vi "Motor Velocity PID.vi"(5 "T_d":dbl=0.01, 6 "DC current max":dbl=0.437, 7 "T_i":dbl=inf, 9 "ccw velocity process variable":dbl[](array[numeric])=[0.0, 0.0, 0.0], 10 "ccw velocity setpoint":dbl[](array[numeric])=[0.0, 0.0, 0.0], 11 "K_p":dbl=0.008) -> (2 "DC current output":dbl[](array[numeric]))   [LabVIEW 2015]
uses:
  <vilib>/Simulation/Implementation/Shared/SIMSCR Execution Mode.ctl
  <vilib>/Simulation/Scripting/Companion Diagram/SimConfigNode/SimParams.ctl
  <vilib>/Simulation/Scripting/Companion Diagram/SimConfigNode/_simSolvers.ctl
  <vilib>/Simulation/Param Hierarchy/Typedefs/SIMPH Param Control Actions.ctl
  <vilib>/Simulation/Implementation/Shared/SIM limit type.ctl
  <vilib>/Simulation/Implementation/Shared/NILVSim_ParamChanged.vi
  <vilib>/Simulation/Implementation/Shared/NILVSIM_BeginStep.vi
  <vilib>/Simulation/ContinuousLinear/Implementation/NILVSim Derivative.llb/SIM derivative (vector).vi
  <vilib>/Simulation/ContinuousLinear/Implementation/NILVSim Integrator new.llb/SIM Integrator Distributor (vector).vi
  <vilib>/Simulation/ContinuousLinear/Implementation/NILVSim Integrator new.llb/SIM Integrator Collector (vector).vi
  <vilib>/Simulation/SignalArithmetic/Implementation/NILVSim Gain.llb/SIM Gain (vector,ScalarGain).vi
  <vilib>/Simulation/Nonlinear/Implementation/NILVSim Saturation.llb/SIM Saturation (vector).vi
  <vilib>/Simulation/Implementation/Shared/NILVSim_Manager.vi
  <vilib>/Utility/error.llb/Clear Errors.vi
  <vilib>/Simulation/Implementation/Shared/NILVSim_FinalizeModel.vi
  <vilib>/Simulation/Implementation/Shared/SIM Unbundle Sim Info.vi
  <vilib>/Simulation/Implementation/Shared/SIMSH Read Queue.vi
  <vilib>/Simulation/Implementation/Shared/NILVSim_Initialize.vi
  <vilib>/Simulation/Utility/Implementation/NILVSim Get Time and IsAcceptedStep.vi
  <vilib>/Simulation/Implementation/Shared/NILVSim_GetModelError.vi
  <vilib>/Simulation/Implementation/Shared/SIM SimErrorHandler.vi
  <vilib>/Simulation/Implementation/Shared/SIM Bundle Sim Info.vi
  <vilib>/Simulation/Scripting/Companion Diagram/SimConfigNode/SimDog.xnode
  <vilib>/Simulation/Implementation/XNodeFramework/SimXNode/SimX.xnode
  <vilib>/Simulation/ContinuousLinear/Implementation/NILVSim Integrator new.llb/SIM Integrator (vector).vi
  <vilib>/Simulation/Implementation/Shared/NI_SIM_Implementation.lvlib
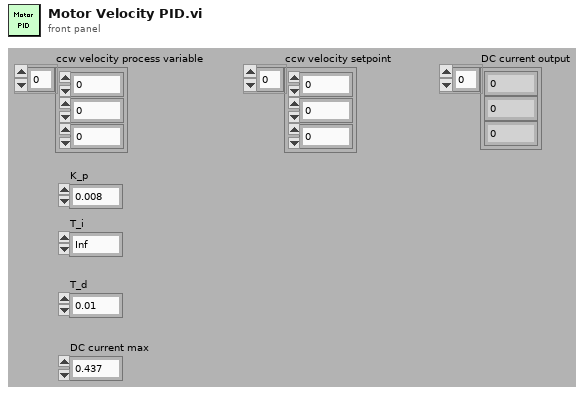
[diagram p1: front panel]
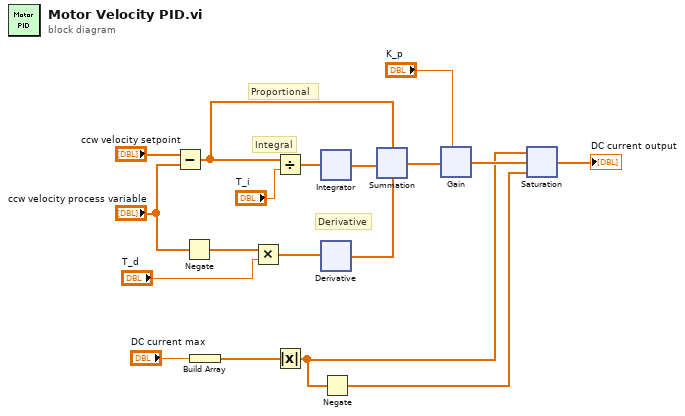
[diagram p0: block diagram]
diagram:
  # "Derivative"
  # "Integral"
  # "Proportional"
  n1 = Subtract(x="ccw velocity setpoint", y="ccw velocity process variable") -> (x-y=w12:dbl[])
  n2 = Negate(x="ccw velocity process variable") -> (-x=w10:dbl[])
  n3 = Build Array("DC current max") -> (w3:dbl[])
  n4 = Multiply(x=w10, y="T_d") -> (x*y=w8:dbl[])
  n5 = Divide(x=w12, y="T_i") -> (x/y=w18:dbl[])
  n6 = Absolute Value(x=w3) -> (abs(x)=w2:dbl[])
  n7 = xnode ("Integrator")("input"=w18) -> ("output"=w16:dbl[])  [unwired: 9 in, 2 out]
  n8 = xnode ("Derivative")("input"=w8) -> ("output"=w7:dbl[])  [unwired: 2 in]
  n9 = Negate ("Negate 2")(x=w2) -> (-x=w1:dbl[])
  n10 = xnode ("Summation")("Operand1"=w12, "Operand2"=w16, "Operand3"=w7) -> ("Result"=w15:dbl[])
  n11 = xnode ("Gain")("gain"="K_p", "input"=w15) -> ("output"=w6:dbl[])  [unwired: 2 in]
  n12 = xnode ("Saturation")("upper limit"=w2, "input"=w6, "lower limit"=w1) -> ("output"=→"DC current output":dbl[])  [unwired: 2 in]
